vi "Check toast done.vi"(6 "Toastiness factor":dbl, 9 "Toastiness Level Set":u8, 10 "Started toasting time":timestamp, 11 "Now":timestamp) -> (3 "Toast done?":bool)   [LabVIEW 2018, in "Toaster.lvlib"]
doc: "Checks whether the total amount of time (set by the toastiness dial) has elapsed."
uses:
  Toaster.lvlib
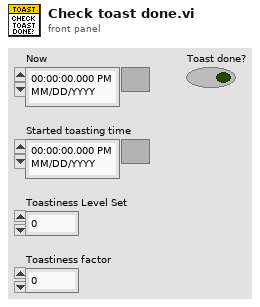
[diagram p1: front panel]
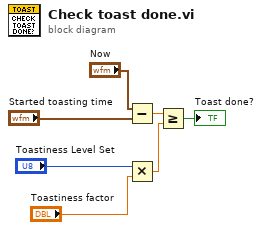
[diagram p0: block diagram]
diagram:
  n1 = Subtract(x="Now", y="Started toasting time") -> (x-y=w6:dbl)
  n2 = Multiply(x="Toastiness Level Set", y="Toastiness factor") -> (x*y=w4:dbl)
  n3 = Greater Or Equal?(x=w6, y=w4) -> (x >= y?=→"Toast done?":bool)
